vi "Drive_Set.vi"   [LabVIEW 2018]
uses:
  Drive_Control_Type.ctl
  <vilib>/Rock Robotics/WPI/DriverStation/WPI_DriverStationRobotMode2.ctl
  Global_Variables/Drive_Globals.vi
  Global_Variables/Robot_Global_Data.vi
  Global_Variables/Sensor_Values.vi
  Global_Variables/Elevator_Globals.vi
  Global_Variables/Climb_Globals.vi
  Global_Variables/Autonomous_Globals.vi
types:
  T1 = typedef "WPI_DriverStationRobotMode2.ctl" = enum16{"Autonomous Disabled", "Autonomous Enabled", "Teleop Disabled", "Teleop Enabled", "Disconnected", "Finish", "Test Disabled", "Test Enabled", "Emergency Stopped"}
  T2 = typedef "Drive_Control_Type.ctl" = enum16{"No_Op", "Write_FL_Position", "Write_FR_Position", "Write_BL_Position", "Write_BR_Position", "Set_Encoder_Positions", "Fieldcentric_PercentVBus", "Fieldcentric", "Robotcentric", "Reset_Gyro", "FR_Wheel", "FL_Wheel", "BR_Wheel", "BL_Wheel", "Drive_Onto_Platform", "Manual_Wheel_Control", "Distance", "Turn_To_Heading", "Turn_To_Target", "Drive_To_Target", "Zero", "Auto_Target", "Drive_Over_Platform", "Heading_Lock", "Time"}
  T3 = typedef "Drive_Notifier.ctl" = cluster{"Drive Control List":T2, "Front/Back":dbl, "Left/Right":dbl, "Turn":dbl, "Test_Joy_Y":dbl, "Test_Joy_X":dbl, "Set Wheel Encoder Positions":bool, "Robotcentric":bool, "Reset Gyro":bool, "Rotate Front Right":bool, "Rotate Front Left":bool, "Rotate Back Right":bool, "Rotate Back Left":bool, "Write_Encoder_Positions":bool, "Climb_Advance":bool, "Parameter_One":dbl, "Parameter_Two":dbl, "Parameter_Three":dbl, "Parameter_Four":dbl, "Drive_Notifier":refnum<notifier>, "Step":i32, "Climb_Reverse":bool, "Auto_Target":bool}
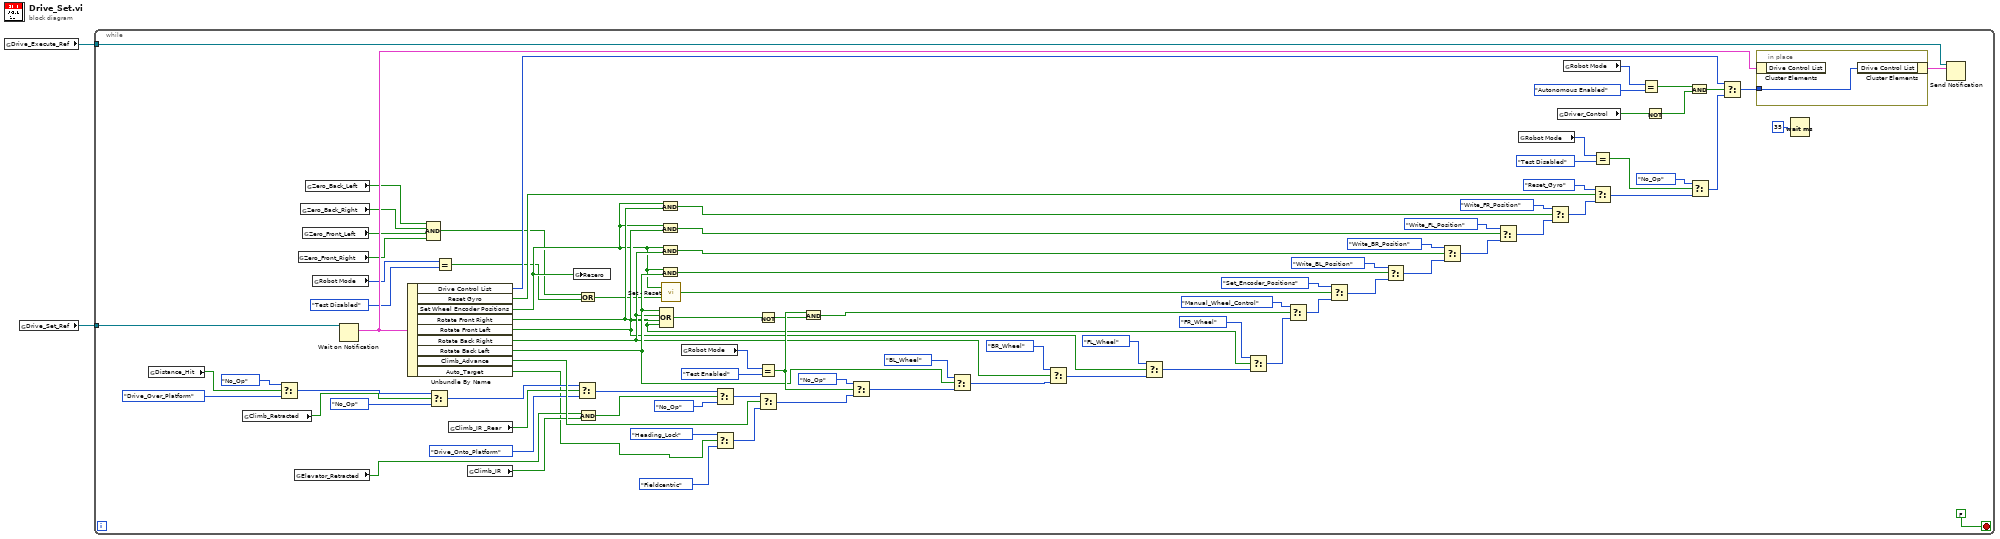
[diagram p0: block diagram]
diagram:
  n1 = global read "Drive_Globals.vi" "Drive_Execute_Ref"() -> (w1:refnum<notifier>)
  n2 = global read "Drive_Globals.vi" "Drive_Set_Ref"() -> (w2:refnum<notifier>)
  n3 = while {
    tunnel: w2 -> [w90]
    tunnel: w1 -> [w80]
    stop <- FALSE stop-if-true
    n4 = global read "Climb_Globals.vi" "Distance_Hit"() -> (w31:bool)
    n5 = global read "Climb_Globals.vi" "Climb_Retracted"() -> (w34:bool)
    n6 = Select(t=Drive_Control_Type."No_Op", s=w31, f=Drive_Control_Type."Drive_Over_Platform") -> (s? t:f=w32:T2)
    n7 = global read "Elevator_Globals.vi" "Elevator_Retracted"() -> (w40:bool)
    n8 = global read "Drive_Globals.vi" "Zero_Front_Right"() -> (w21:bool)
    n9 = global read "Drive_Globals.vi" "Zero_Back_Right"() -> (w19:bool)
    n10 = global read "Drive_Globals.vi" "Zero_Front_Left"() -> (w20:bool)
    n11 = global read "Drive_Globals.vi" "Zero_Back_Left"() -> (w18:bool)
    n12 = global read "Robot_Global_Data.vi" "Robot Mode"() -> (w12:T1)
    n13 = Wait on Notification(notifier=w90) -> (notification=w89:T3)  [unwired: 3 in, 3 out]
    n14 = Unbundle By Name(w89) -> ("Drive Control List"=w71:T2, "Reset Gyro"=w88:bool, "Set Wheel Encoder Positions"=w24:bool, "Rotate Front Right"=w48:bool, "Rotate Front Left"=w49:bool, "Rotate Back Right"=w50:bool, "Rotate Back Left"=w51:bool, "Climb_Advance"=w43:bool, "Auto_Target"=w3:bool)
    n15 = Compound Arithmetic op=AND(w18, w19, w20, w21) -> (w9:bool)
    n16 = Select(t=w32, s=w34, f=Drive_Control_Type."No_Op") -> (s? t:f=w35:T2)
    n17 = Equal?(x=w12, y=WPI_DriverStationRobotMode2."Test Disabled") -> (x = y?=w10:bool)
    n18 = global read "Sensor_Values.vi" "Climb_IR _Rear"() -> (w37:bool)
    n19 = global read "Sensor_Values.vi" "Climb_IR"() -> (w39:bool)
    n20 = global write "Sensor_Values.vi" "Rezero"(w24) -> ()
    n21 = Select(t=w35, s=w37, f=Drive_Control_Type."Drive_Onto_Platform" ("t")) -> (s? t:f=w38:T2)
    n22 = Or(x=w9, y=w10) -> (x .or. y?=w8:bool)
    n23 = And(x=w40, y=w39) -> (x .and. y?=w41:bool)
    n24 = Compound Arithmetic op=OR(w51, w50, w49, w48) -> (w67:bool)
    n25 = And(x=w24, y=w48) -> (x .and. y?=w59:bool)
    n26 = And(x=w24, y=w49) -> (x .and. y?=w58:bool)
    n27 = And(x=w24, y=w50) -> (x .and. y?=w57:bool)
    n28 = And(x=w24, y=w51) -> (x .and. y?=w56:bool)
    n29 = call "Set - Reset.vi"("Reset"=w8, "Set"=w24) -> ("Output"=w25:bool)
    n30 = global read "Robot_Global_Data.vi" "Robot Mode"() -> (w83:T1)
    n31 = Select(t=w38, s=w41, f=Drive_Control_Type."No_Op" ("t")) -> (s? t:f=w42:T2)
    n32 = Select(t=Drive_Control_Type."Heading_Lock", s=w3, f=Drive_Control_Type."Fieldcentric") -> (s? t:f=w28:T2)
    n33 = Not(x=w67) -> (.not. x?=w26:bool)
    n34 = Equal?(x=w83, y=WPI_DriverStationRobotMode2."Test Enabled") -> (x = y?=w65:bool)
    n35 = Select(t=w42, s=w43, f=w28) -> (s? t:f=w47:T2)
    n36 = And(x=w65, y=w26) -> (x .and. y?=w66:bool)
    n37 = Select(t=Drive_Control_Type."No_Op", s=w65, f=w47) -> (s? t:f=w81:T2)
    n38 = Select(t=Drive_Control_Type."BL_Wheel", s=w51, f=w81) -> (s? t:f=w84:T2)
    n39 = Select(t=Drive_Control_Type."BR_Wheel", s=w50, f=w84) -> (s? t:f=w85:T2)
    n40 = Select(t=Drive_Control_Type."FL_Wheel", s=w49, f=w85) -> (s? t:f=w86:T2)
    n41 = Select(t=Drive_Control_Type."FR_Wheel" ("f"), s=w48, f=w86) -> (s? t:f=w70:T2)
    n42 = Select(t=Drive_Control_Type."Manual_Wheel_Control", s=w66, f=w70) -> (s? t:f=w69:T2)
    n43 = Select(t=Drive_Control_Type."Set_Encoder_Positions" ("f"), s=w25, f=w69) -> (s? t:f=w64:T2)
    n44 = Select(t=Drive_Control_Type."Write_BL_Position", s=w56, f=w64) -> (s? t:f=w62:T2)
    n45 = Select(t=Drive_Control_Type."Write_BR_Position", s=w57, f=w62) -> (s? t:f=w61:T2)
    n46 = Select(t=Drive_Control_Type."Write_FL_Position", s=w58, f=w61) -> (s? t:f=w60:T2)
    n47 = global read "Robot_Global_Data.vi" "Robot Mode"() -> (w22:T1)
    n48 = Select(t=Drive_Control_Type."Write_FR_Position", s=w59, f=w60) -> (s? t:f=w63:T2)
    n49 = global read "Autonomous_Globals.vi" "Driver_Control"() -> (w6:bool)
    n50 = global read "Robot_Global_Data.vi" "Robot Mode"() -> (w72:T1)
    n51 = Equal?(x=w22, y=WPI_DriverStationRobotMode2."Test Disabled") -> (x = y?=w16:bool)
    n52 = Select(t=Drive_Control_Type."Reset_Gyro", s=w88, f=w63) -> (s? t:f=w14:T2)
    n53 = Equal?(x=w72, y=WPI_DriverStationRobotMode2."Autonomous Enabled") -> (x = y?=w5:bool)
    n54 = Not(x=w6) -> (.not. x?=w7:bool)
    n55 = And(x=w5, y=w7) -> (x .and. y?=w4:bool)
    n56 = Select(t=Drive_Control_Type."No_Op" ("f"), s=w16, f=w14) -> (s? t:f=w13:T2)
    n57 = Select(t=w71, s=w4, f=w13) -> (s? t:f=w45:T2)
    n58 = in-place {
      in-place-border: w45 -> [w93]
      n59 = in-place-cluster #1(w89) -> ()  [unwired: 1 out]
      n60 = in-place-cluster #1("Drive Control List"=w93) -> (w79:T3)
    }
    n61 = Wait (ms)(milliseconds to wait=u32 35) -> ()  [unwired: 1 out]
    n62 = Send Notification(notification=w79, notifier=w80) -> ()  [unwired: 1 in, 2 out]
  }
